vi "Create All Message Queues.vi"(8 "error in (no error)":errorcluster) -> (0 "error out":errorcluster, 3 "Message Queues out":T1)   [LabVIEW 2020, in "Message Queue.lvlib"]
uses:
  Message Queue.lvlib
  All Message Queues.ctl
  Message Cluster.ctl
  Enqueue Message (Single).vi
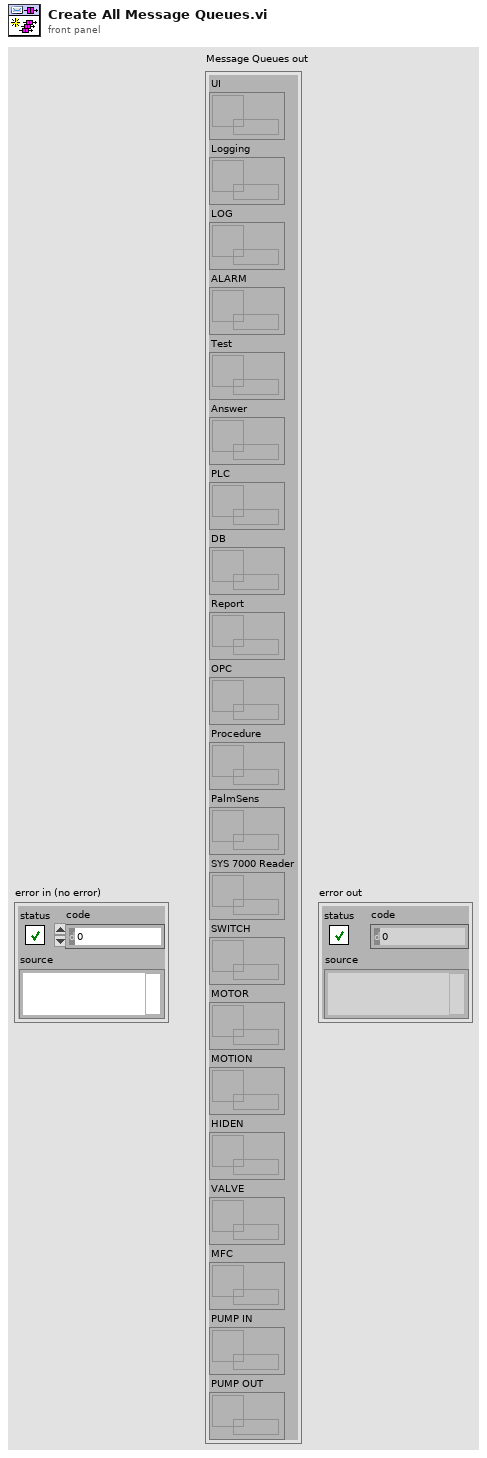
[diagram p1: front panel]
types:
  T1 = typedef "Message Queue.lvlib/All Message Queues.ctl" = cluster{"UI":refnum<queue>, "Logging":refnum<queue>, "LOG":refnum<queue>, "ALARM":refnum<queue>, "Test":refnum<queue>, "Answer":refnum<queue>, "PLC":refnum<queue>, "DB":refnum<queue>, "Report":refnum<queue>, "OPC":refnum<queue>, "Procedure":refnum<queue>, "PalmSens":refnum<queue>, "SYS 7000 Reader":refnum<queue>, "SWITCH":refnum<queue>, "MOTOR":refnum<queue>, "MOTION":refnum<queue>, "HIDEN":refnum<queue>, "VALVE":refnum<queue>, "MFC":refnum<queue>, "PUMP IN":refnum<queue>, "PUMP OUT":refnum<queue>}
  T2 = cluster{"[0]":refnum<queue>, "[1]":refnum<queue>, "[2]":refnum<queue>, "[3]":refnum<queue>, "[4]":refnum<queue>, "[5]":refnum<queue>, "[6]":refnum<queue>, "[7]":refnum<queue>, "[8]":refnum<queue>, "[9]":refnum<queue>, "[10]":refnum<queue>, "[11]":refnum<queue>, "[12]":refnum<queue>, "[13]":refnum<queue>, "[14]":refnum<queue>, "[15]":refnum<queue>, "[16]":refnum<queue>, "[17]":refnum<queue>, "[18]":refnum<queue>, "[19]":refnum<queue>, "[20]":refnum<queue>}
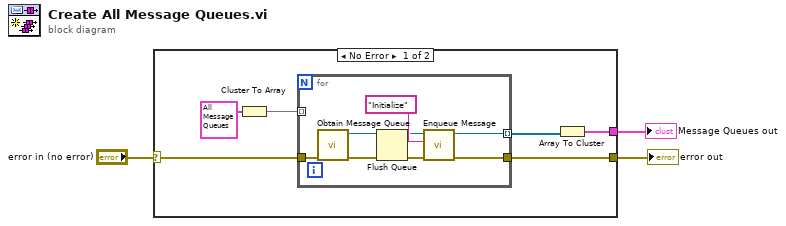
[diagram p0: block diagram]
diagram:
  n1 = case shown="No Error" "error in (no error)" {
    selector: "error in (no error)" -> [w9 w17]
    tunnel: [w8 w17] -> w3
    tunnel: [w7 _] -> w2
    frame No Error {
      n2 = Cluster To Array(cluster=T1 {"UI"=refnum, "Logging"=refnum, "LOG"=refnum, "ALARM"=refnum, "Test"=refnum, "Answer"=refnum, "PLC"=refnum, "DB"=refnum, "Report"=refnum, "OPC"=refnum, "Procedure"=refnum, "PalmSens"=refnum, "SYS 7000 Reader"=refnum, "SWITCH"=refnum, "MOTOR"=refnum, "MOTION"=refnum, "HIDEN"=refnum, "VALVE"=refnum, "MFC"=refnum, "PUMP IN"=refnum, "PUMP OUT"=refnum} ("Message Queues out")) -> (array=w4:refnum<queue>[])
      n3 = for {
        tunnel: [w12] -> w6 mode=indexing
        tunnel: w4 -> [_] mode=indexing
        tunnel: w9 -> [w14]
        tunnel: [w11] -> w8
        n4 = call "Obtain Message Queue.vi"("error in (no error)"=w14) -> ("error out"=w16:errorcluster, "Message Queue"=w15:refnum<queue>)  [unwired: 9 in]
        n5 = Flush Queue(queue=w15) -> (queue out=w10:refnum<queue>)  [unwired: 1 in, 2 out]
        n6 = call-poly "Enqueue Message.vi"("error in (no error)"=w16, "Message"="Initialize", "Message Queue"=w10) -> ("error out"=w11:errorcluster, "dup Message Queue"=w12:refnum<queue>)  [unwired: 7 in]
      }
      n7 = Array To Cluster(array=w6) -> (cluster=w7:T2)
    }
    frame Error {
    }
  }
  "Message Queues out" <- w2
  "error out" <- w3
